vi "DAQmx(AI).SetTDMSLogFile.vi"(8 "error in (no error)":errorcluster, 9 "Group Name":string, 10 "TDMS File Path":path, 11 "DAQmx(AI) in":refnum<class "DAQmx(AI).lvclass">) -> (0 "error out":errorcluster, 3 "DAQmx(AI) out":refnum<class "DAQmx(AI).lvclass">)   [LabVIEW 2019, in "DAQmx(AI).lvclass"]
uses:
  DAQmx(AI).lvclass
  DAQmx(AI).lvclass/DAQmx(AI).ctl
  <vilib>/DAQmx/configure/task.llb/DAQmx Configure Logging (TDMS).vi
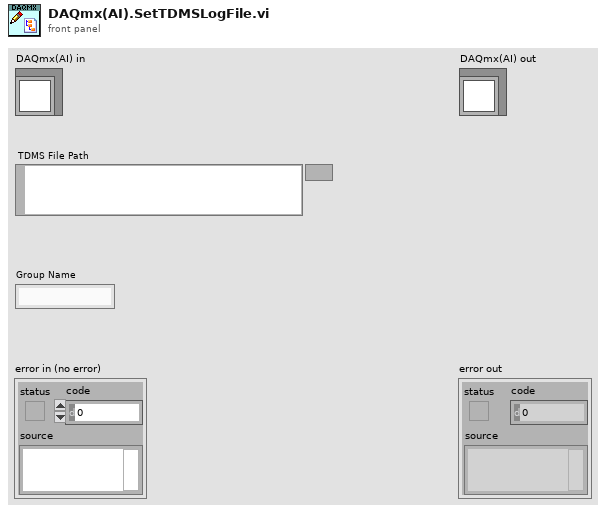
[diagram p1: front panel]
types:
  T1 = typedef "DAQmx(AI).lvclass/PrivateData--Ref.ctl" = refnum<data-value>
  T2 = typedef "DAQmx(AI).lvclass/PrivateData--Cluster.ctl" = cluster{"Configuration":T3, "Public Events":T5, "Data":dbl, "Scaling":T6, "Private Events":T12}
  T3 = typedef "DAQmx(AI).lvclass/Configuration--Cluster.ctl" = cluster{"PhysChan":tag, "Period (ms)":i64, "input terminal cfg":i32, "minimum value":dbl, "maximum value":dbl, "units":T4, "task name":string, "TDMS File Path":path, "Group Name":string}
  T4 = typedef "DAQmx(AI).lvclass/Units -- Enum.ctl" = enum16{"Volts", "Amps", "Deg F", "Deg C", "Deg R", "Kelvins", "Strain", "Ohms", "Hz", "Seconds", "Meters", "Inches", "Degrees", "Radians", "Ticks", "g", "m/s^2", "m/s", "in/s", "Pascals", "Newtons", "Pounds", "kgf", "psi", "bar", "Nm", "oz-in", "lb-in", "lb-ft", "Volts/Volt", "mVolts/Volt", "From TEDS"}
  T5 = typedef "DAQmx(AI).lvclass/PublicEvents--Cluster.ctl" = cluster{"Value Changed":refnum<user-event>, "Task Configuration":refnum<user-event>, "Scaling":refnum<user-event>}
  T6 = typedef "DAQmx(AI).lvclass/Scaling--Cluster.ctl" = cluster{"Scale Name":string, "Scale Type":T7, "Scaled Units":string, "Linear":T8, "Map Range":T9, "Polynomial":T10, "Table":T11}
  T7 = typedef "DAQmx(AI).lvclass/ScalingType--Enum.ctl" = enum16{"No scaling", "Linear", "Map Range", "Polynomial", "Table"}
  T8 = typedef "DAQmx(AI).lvclass/Scaling(Linear)--Cluster.ctl" = cluster{"Slope":dbl, "Intercept":dbl}
  T9 = typedef "DAQmx(AI).lvclass/Scaling(MapRange)--Cluster.ctl" = cluster{"Minimum":dbl, "Maximum":dbl}
  T10 = typedef "DAQmx(AI).lvclass/Scaling(Polynomial)--Cluster.ctl" = cluster{"forward coeff":dbl[], "reverse coeff":dbl[]}
  T11 = typedef "DAQmx(AI).lvclass/Scaling(Table)--Cluster.ctl" = cluster{"scaled values":dbl[], "pres-scaled values":dbl[]}
  T12 = typedef "DAQmx(AI).lvclass/PrivateEvents--Cluster.ctl" = cluster{"Logging":refnum<user-event>}
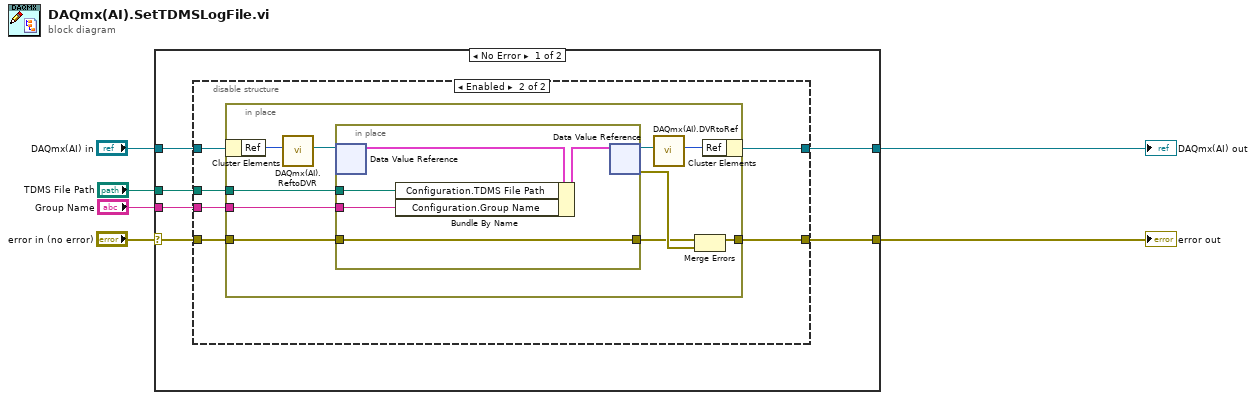
[diagram p0: block diagram]
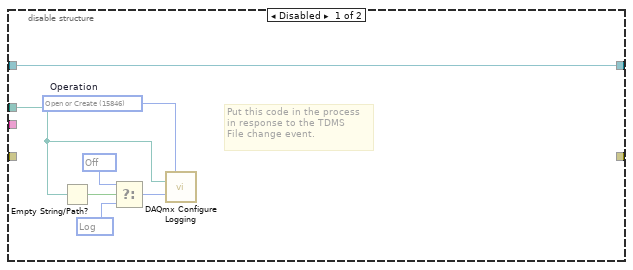
[diagram p2: hidden frame]
diagram:
  n1 = case shown="No Error" "error in (no error)" {
    selector: "error in (no error)" -> [w8 w42]
    tunnel: [w7 w42] -> w5
    tunnel: [w10 w41] -> w3
    tunnel: "DAQmx(AI) in" -> [w11 w41]
    tunnel: "TDMS File Path" -> [w12 _]
    tunnel: "Group Name" -> [w9 _]
    frame No Error {
      n2 = disable-structure shown="Enabled" {
        disable-tunnel: w12 -> [w14 w21]
        disable-tunnel: [w13 w24] -> w10
        disable-tunnel: w11 -> [w13 w25]
        disable-tunnel: w9 -> [_ w20]
        disable-tunnel: w8 -> [_ w23]
        disable-tunnel: [_ w22] -> w7
        frame Disabled {
          w15 = 10231 items=["Off"=10231, "Log"=15844, "Log and Read"=15842] ("logging mode")
          w17 = 15844 items=["Off"=10231, "Log"=15844, "Log and Read"=15842] ("logging mode")
          w19 = 15846 items=["Open"=10437, "Open or Create"=15846, "Create or Replace"=15847, "Create"=15848]  # Operation
          # "Put this code in the process\nin response to the TDMS\nFile change event."
          n3 = Empty String/Path?(string/path=w14) -> (empty?=w18:bool)
          n4 = Select(t=w15, s=w18, f=w17) -> (s? t:f=w16:i32)
          n5 = call-poly <vilib>:"DAQmx Configure Logging.vi"("operation"=w19, "file path"=w14, "logging mode"=w16) -> ()  [unwired: 11 in, 2 out]
        }
        frame Enabled {
          n6 = in-place {
            in-place-border: w23 -> [w35]
            in-place-border: [w32] -> w22
            in-place-border: w21 -> [w27]
            in-place-border: w20 -> [w26]
            n7 = in-place-cluster #1(w25) -> ("Ref"=w31:u32)
            n8 = call "DAQmx(AI).ReftoDVR.vi"("Ref"=w31) -> ("Ref"=w30:T1)  [unwired: 10 in]
            n9 = in-place {
              in-place-border: w35 -> [w40]
              in-place-border: [w40] -> w33
              in-place-border: w27 -> [w37]
              in-place-border: w26 -> [w36]
              n10 = in-place-dvr #2(w30) -> (w39:T2)  [unwired: 1 out]
              n11 = Bundle By Name(cluster=w39, "Configuration.TDMS File Path"=w37, "Configuration.Group Name"=w36) -> (w38:T2)
              n12 = in-place-dvr #2(w38) -> (w29:T1, w34:errorcluster)
            }
            n13 = call "DAQmx(AI).DVRtoRef.vi"("Ref"=w29) -> ("Ref"=w28:u32)  [unwired: 10 in]
            n14 = Merge Errors(w33, w34) -> (w32:errorcluster)
            n15 = in-place-cluster #1("Ref"=w28) -> (w24:refnum<class "DAQmx(AI).lvclass">)
          }
        }
      }
    }
    frame Error {
    }
  }
  "error out" <- w5
  "DAQmx(AI) out" <- w3
